vi "WriteDataFifo.vi"(8 "error in (no error)":errorcluster, 10 "PmuReport":T1 {"Synx" format="%#_4g"}, 11 "PmuBase in":refnum<class "PmuBase.lvclass">) -> (0 "error out":errorcluster, 3 "PmuBase out":refnum<class "PmuBase.lvclass">)   [LabVIEW 2018, in "SensorPlugins.lvlib" / "PmuBase.lvclass"]
uses:
  PmuBase.lvclass
  C:/Users/ico/Documents/Projects/NistPluggableModules/Sensor/SensorPlugins/SensorBaseClass/SensorBase.lvclass
  Typedef/PmuData.ctl
  PmuBase.lvclass/PmuBase.ctl
  Accessors/Read PmuDataArray.vi
  Accessors/Read DataFifo.vi
  Accessors/Write PmuDataArray.vi
  Accessors/Write DataFifo.vi
  <vilib>/Utility/error.llb/Error Cluster From Error Code.vi
  <vilib>/ErrorRing/Error Ring.xnode
  SensorPlugins.lvlib
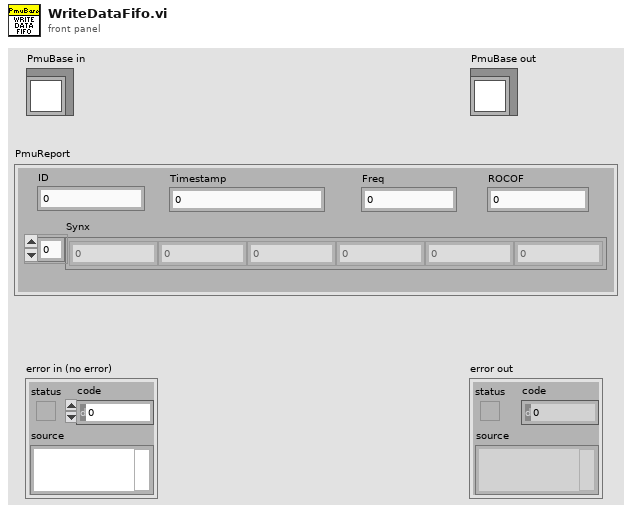
[diagram p1: front panel]
types:
  T1 = typedef "SensorPlugins.lvlib/PmuBase.lvclass/PmuData.ctl" = cluster{"Timestamp":dbl, "Synx":cdb[], "Freq":dbl, "ROCOF":dbl, "ID":i16}
  T2 = typedef "DataFifo.ctl" = cluster{"ReadPointer":u16, "WritePointer":u64, "Locked":bool, "FifoSize":u64}
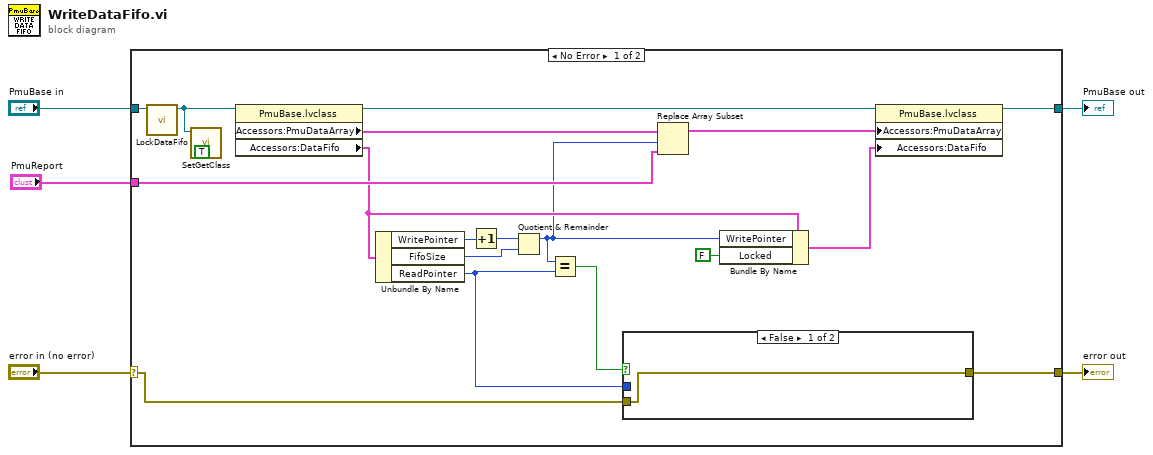
[diagram p0: block diagram]
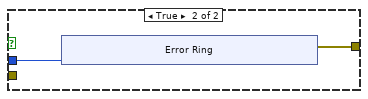
[diagram p2: hidden frame]
diagram:
  n1 = case shown="No Error" "error in (no error)" {
    selector: "error in (no error)" -> [w8 w36]
    tunnel: [w17 w36] -> w4
    tunnel: [w14 w35] -> w2
    tunnel: "PmuBase in" -> [w24 w35]
    tunnel: "PmuReport" -> [w15 _]
    frame No Error {
      n2 = call "LockDataFifo.vi"("PmuBase in"=w24) -> ("PmuBase out"=w23:refnum<class "PmuBase.lvclass">)  [unwired: 9 in, 1 out]
      n3 = call "SetGetClass.vi"("Set (f)"=TRUE, "Class In"=w23) -> ()  [unwired: 9 in, 1 out]
      n4 = property class="PmuBase.lvclass"(reference=w23) -> (reference out=w21:refnum<class "PmuBase.lvclass">, "Accessors:PmuDataArray"=w16:T1[], "Accessors:DataFifo"=w13:T2)  [unwired: 1 in, 1 out]
      n5 = Unbundle By Name(w13) -> ("WritePointer"=w20:u64, "FifoSize"=w6:u64, "ReadPointer"=w7:u16)
      n6 = Increment(x=w20) -> (x+1=w19:u64)
      n7 = Quotient & Remainder(x=w19, y=w6) -> (x-y*floor(x/y)=w12:u64)  [unwired: 1 out]
      n8 = Equal?(x=w12, y=w7) -> (x = y?=w18:bool)
      n9 = case shown="False" w18 {
        tunnel: w7 -> [_ w27]
        tunnel: [w25 w26] -> w17
        tunnel: w8 -> [w25 _]
        frame False {
        }
        frame True {
          n10 = xnode "Error Ring"("parameter 0"=w27) -> ("error out"=w26:errorcluster)
        }
      }
      n11 = Replace Array Subset(array=w16, new element=w15, index=w12) -> (w9:T1[])
      n12 = Bundle By Name(cluster=w13, "WritePointer"=w12, "Locked"=FALSE) -> (w10:T2)
      n13 = property class="PmuBase.lvclass"(reference=w21, "Accessors:PmuDataArray"=w9, "Accessors:DataFifo"=w10) -> (reference out=w14:refnum<class "PmuBase.lvclass">)  [unwired: 1 in, 1 out]
    }
    frame Error {
    }
  }
  "error out" <- w4
  "PmuBase out" <- w2
